vi "json_error.vi"(0 "m":string, 5 "text":string, 9 "at":i32) -> (15 "error out":errorcluster)   [LabVIEW 2011]
doc: "Format an error."
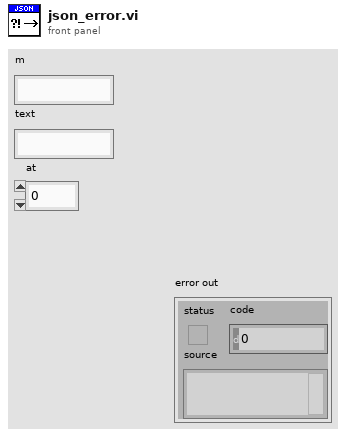
[diagram p1: front panel]
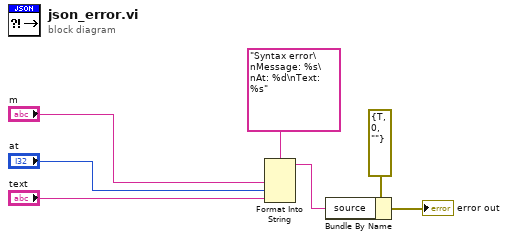
[diagram p0: block diagram]
diagram:
  n1 = Format Into String(format string="Syntax error\nMessage: %s\nAt: %d\nText: %s", "m", "at", "text") -> (resulting string=w2:string)  [unwired: 2 in, 1 out]
  n2 = Bundle By Name(cluster=errorcluster {"status"=TRUE, "code"=0, "source"=""} ("error out"), "source"=w2) -> (→"error out":errorcluster)
